vi "MongoDB.GetCreate_Collection.vi"(8 "error in (no error)":errorcluster, 10 "collectionName":string, 11 "MongoDB.Database in":refnum<class "MongoDB.Database.lvclass">) -> (0 "error out":errorcluster, 2 "MongoDB.Collection out":refnum<class "MongoDB.Collection.lvclass">, 3 "MongoDB.Database out":refnum<class "MongoDB.Database.lvclass">)   [LabVIEW 2014, in "MongoDB.Database.lvclass"]
uses:
  MongoDB.Database.lvclass
  MongoDB.Collection.lvclass
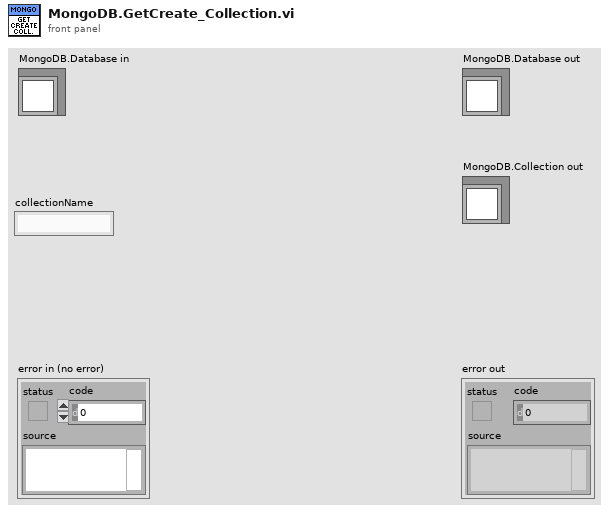
[diagram p1: front panel]
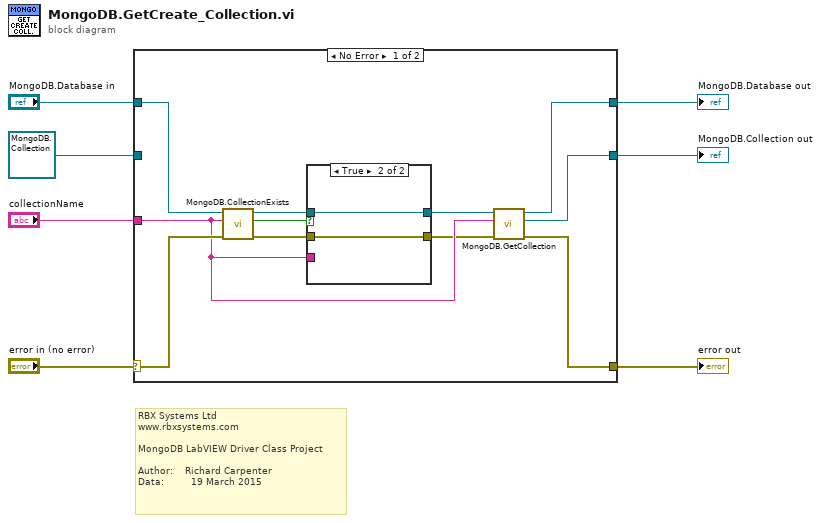
[diagram p0: block diagram]
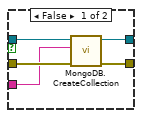
[diagram p2: hidden frame]
diagram:
  # "RBX Systems Ltd\nwww.rbxsystems.com\n\nMongoDB LabVIEW Driver Class Project\n\nAuthor:    Richard Carpenter\nData:         19 March 2015"
  n1 = case shown="No Error" "error in (no error)" {
    selector: "error in (no error)" -> [w17 w28]
    tunnel: [w10 w28] -> w6
    tunnel: [w8 w27] -> w4
    tunnel: "MongoDB.Database in" -> [w18 w27]
    tunnel: [w9 w26] -> w3
    tunnel: refnum<class "MongoDB.Collection.lvclass"> refnum ("MongoDB.Collection in") -> [_ w26]
    tunnel: "collectionName" -> [w12 _]
    frame No Error {
      n2 = call-dynamic "MongoDB.CollectionExists.vi"("error in (no error)"=w17, "collectionName"=w12, "MongoDB.Database in"=w18) -> ("error out"=w14:errorcluster, "CollectionExists"=w16:bool, "MongoDB.Database out"=w15:refnum<class "MongoDB.Database.lvclass">)  [unwired: 6 in]
      n3 = case shown="True" w16 {
        tunnel: w15 -> [w23 w25]
        tunnel: w14 -> [w22 w24]
        tunnel: w12 -> [w21 _]
        tunnel: [w20 w25] -> w13
        tunnel: [w19 w24] -> w11
        frame False {
          n4 = call "MongoDB.CreateCollection.vi"("error in (no error)"=w22, "collectionName"=w21, "MongoDB.Database in"=w23) -> ("error out"=w19:errorcluster, "MongoDB.Database out"=w20:refnum<class "MongoDB.Database.lvclass">)  [unwired: 6 in, 1 out]
        }
        frame True {
        }
      }
      n5 = call "MongoDB.GetCollection.vi"("error in (no error)"=w11, "collectionName"=w12, "MongoDB.Database in"=w13) -> ("error out"=w10:errorcluster, "MongoDB.Collection out"=w9:refnum<class "MongoDB.Collection.lvclass">, "MongoDB.Database out"=w8:refnum<class "MongoDB.Database.lvclass">)  [unwired: 6 in]
    }
    frame Error {
    }
  }
  "error out" <- w6
  "MongoDB.Database out" <- w4
  "MongoDB.Collection out" <- w3
